vi "Parse Labels in Channel.vi"(8 "error in":errorcluster, 9 "channel #":u16, 10 "direction":T1, 11 "node in":refnum<k20>) -> (0 "error out":errorcluster, 3 "labels":T2[](array[typedef]))   [LabVIEW 2020, in "ARINC 429 Import.lvlib"]
uses:
  ARINC 429 Import.lvlib
  Encoding and Decoding/Encoding.ctl
  Encoding and Decoding/Encoding and Decoding.lvlib
  Read Tag Element (Boolean).vi
  Shared/Parameter Definition.ctl
  Shared/Direction.ctl
  Shared/VS Channel Definition for Parameter.ctl
  Shared/VS Channels Definition for Label.ctl
  Shared/Transfer Type.ctl
  Read Tag Element (String).vi
  Read Tag Element (U16).vi
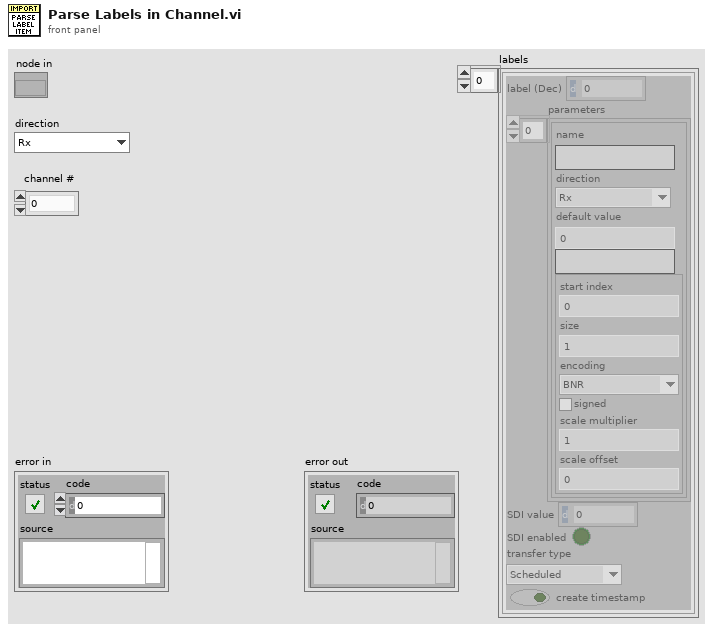
[diagram p1: front panel]
types:
  T1 = typedef "Direction.ctl" = enum16{"Rx", "Tx"}
  T2 = typedef "VS Channels Definition for Label.ctl" = cluster{"label (Dec)":u32, "parameters":T3[], "SDI value":u8, "SDI enabled":bool, "transfer type":T6, "create timestamp":bool}
  T3 = typedef "VS Channel Definition for Parameter.ctl" = cluster{"name":string, "direction":T1, "default value":dbl, "unit":string, "Parameter":T4}
  T4 = typedef "Parameter Definition.ctl" = cluster{"start index":i32, "size":i32, "encoding":T5, "signed":bool, "scale multiplier":dbl, "scale offset":dbl}
  T5 = typedef "Encoding and Decoding.lvlib/Encoding.ctl" = enum16{"BNR", "BCD", "Discrete"}
  T6 = typedef "Transfer Type.ctl" = enum16{"Scheduled", "Acyclic", "Block", "Strobe"}
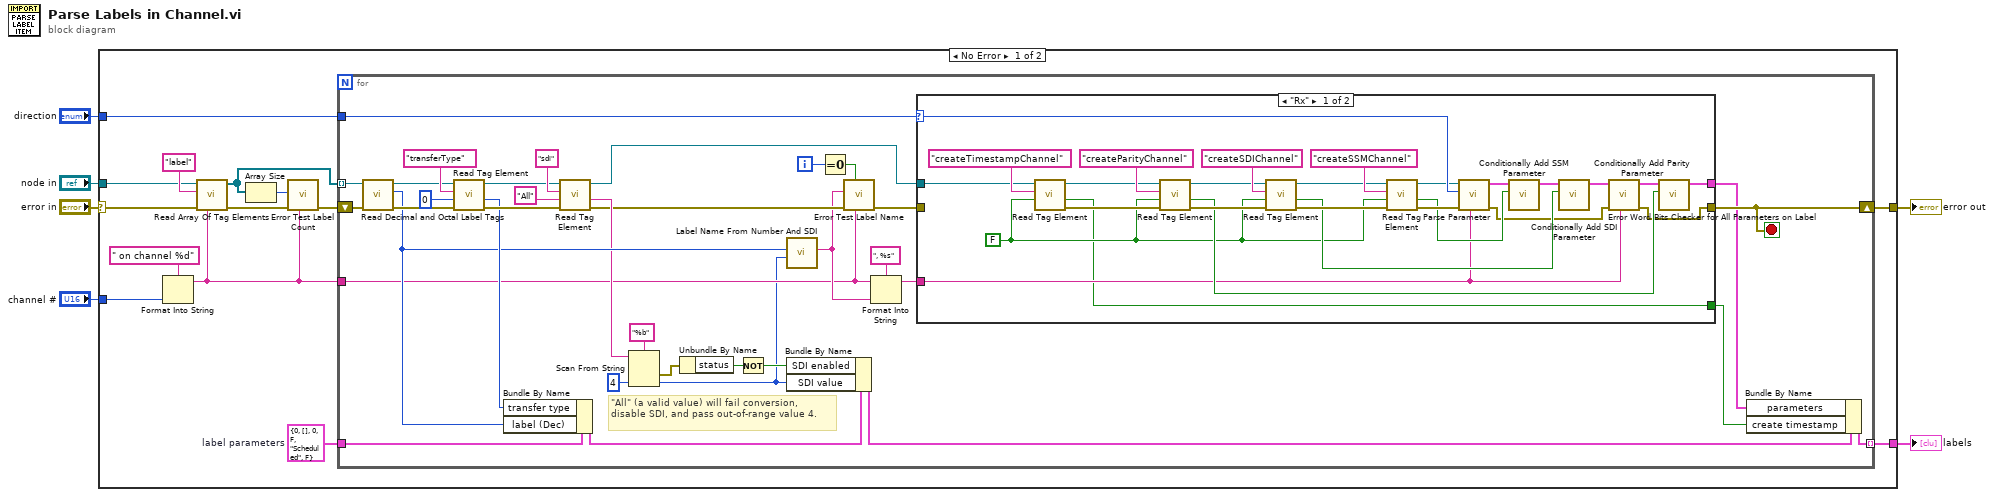
[diagram p0: block diagram]
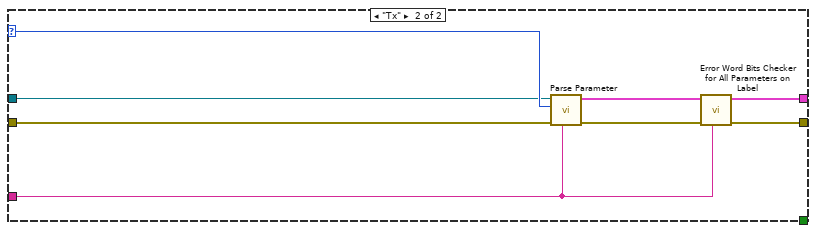
[diagram p2: hidden frame]
diagram:
  n1 = case shown="No Error" "error in" {
    selector: "error in" -> [w13 w92]
    tunnel: [w20 _] -> w6
    tunnel: "node in" -> [w16 _]
    tunnel: [w15 w92] -> w4
    tunnel: "direction" -> [w14 _]
    tunnel: "channel #" -> [w9 _]
    frame No Error {
      w11 = T2 {"label (Dec)"=0, "parameters"=[], "SDI value"=0, "SDI enabled"=FALSE, "transfer type"=enum."Scheduled", "create timestamp"=FALSE}  # label parameters
      n2 = Format Into String(format string=" on channel %d", w9) -> (resulting string=w10:string)  [unwired: 2 in, 1 out]
      n3 = call "Read Array Of Tag Elements.vi"("error text in"=w10, "error in"=w13, "tag name"="label" ("Tag Name"), "node in"=w16) -> ("error out"=w18:errorcluster, "array of elements"=w7:refnum<k20>[])  [unwired: 6 in]
      n4 = Array Size(array=w7) -> (size(s)=w8:i32)
      n5 = call "Error Test Label Count.vi"("error text in"=w10, "error in"=w18, "number of labels"=w8) -> ("error out"=w17:errorcluster)  [unwired: 8 in]
      n6 = for {
        shift-right: [w34] -> w15
        shift-left: w17 -> [w37]
        tunnel: [w48] -> w20 mode=indexing
        tunnel: w7 -> [w46] mode=indexing
        tunnel: w14 -> [w35]
        tunnel: w11 -> [w38]
        tunnel: w10 -> [w23]
        i -> [w26]
        stop <- w34 stop-if-true
        # "\"All\" (a valid value) will fail conversion, disable SDI, and pass out-of-range value 4."
        n7 = call "Read Decimal and Octal Label Tags.vi"("error in"=w37, "node in"=w46) -> ("error out"=w43:errorcluster, "label (Dec)"=w31:u32, "node out"=w44:refnum<k20>)  [unwired: 7 in]
        n8 = call-poly "Read Tag Element.vi"("error in"=w43, "default"=u16 0, "Tag Name"="transferType", "node in"=w44) -> ("error out"=w41:errorcluster, "value"=w39:u16, "node out"=w42:refnum<k20>)  [unwired: 5 in]
        n9 = Bundle By Name(cluster=w38, "transfer type"=w39, "label (Dec)"=w31) -> (w47:T2)
        n10 = call-poly "Read Tag Element.vi"("error in"=w41, "default"="All", "Tag Name"="sdi", "node in"=w42) -> ("error out"=w29:errorcluster, "value"=w30:string, "node out"=w27:refnum<k20>)  [unwired: 5 in]
        n11 = Scan From String(format string="%b", input string=w30, default 1=u8 4 ("default value 1")) -> (error out=w52:errorcluster, output 1=w22:u8)  [unwired: 2 in, 2 out]
        n12 = Unbundle By Name(w52) -> ("status"=w51:bool)
        n13 = Not(x=w51) -> (.not. x?=w50:bool)
        n14 = call "Label Name From Number And SDI.vi"("SDI value"=w22, "label (Dec)"=w31) -> ("label name"=w24:string)  [unwired: 9 in]
        n15 = Bundle By Name(cluster=w47, "SDI enabled"=w50, "SDI value"=w22) -> (w49:T2)
        n16 = Equal To 0?(x=w26) -> (x = 0?=w25:bool)
        n17 = call "Error Test Label Name.vi"("error text in"=w23, "reset (F)"=w25, "error in"=w29, "label name"=w24) -> ("error out"=w28:errorcluster)  [unwired: 7 in]
        n18 = Format Into String(format string=", %s", initial string=w23, w24) -> (resulting string=w33:string)  [unwired: 1 in, 1 out]
        n19 = case shown="\"Rx\"" w35 {
          selector: w35 -> [w77 w91]
          tunnel: [w64 w89] -> w34
          tunnel: w33 -> [w63 w84]
          tunnel: [w75 w88] -> w32
          tunnel: w27 -> [w61 w87]
          tunnel: w28 -> [_ w86]
          tunnel: [w57 _] -> w21
          frame "Rx" {
            w58 = FALSE
            n20 = call-poly "Read Tag Element.vi"("default"=w58, "Tag Name"="createTimestampChannel", "node in"=w61) -> ("error out"=w59:errorcluster, "value"=w57:bool, "node out"=w60:refnum<k20>)  [unwired: 6 in]
            n21 = call-poly "Read Tag Element.vi"("error in"=w59, "default"=w58, "Tag Name"="createParityChannel", "node in"=w60) -> ("error out"=w73:errorcluster, "value"=w67:bool, "node out"=w74:refnum<k20>)  [unwired: 5 in]
            n22 = call-poly "Read Tag Element.vi"("error in"=w73, "default"=w58, "Tag Name"="createSDIChannel", "node in"=w74) -> ("error out"=w79:errorcluster, "value"=w78:bool, "node out"=w80:refnum<k20>)  [unwired: 5 in]
            n23 = call-poly "Read Tag Element.vi"("error in"=w79, "default"=w58, "Tag Name"="createSSMChannel", "node in"=w80) -> ("error out"=w71:errorcluster, "value"=w66:bool, "node out"=w72:refnum<k20>)  [unwired: 5 in]
            n24 = call "Parse Parameter.vi"("error text in"=w63, "error in"=w71, "direction"=w77, "node in"=w72) -> ("error out"=w65:errorcluster, "parametesrs"=w70:T3[])  [unwired: 6 in]
            n25 = call "Conditionally Add SSM Parameter.vi"("create SSM (F)"=w66, "parameters in"=w70) -> ("parameters out"=w69:T3[])  [unwired: 9 in]
            n26 = call "Conditionally Add SDI Parameter.vi"("create SDI (F)"=w78, "parameters in"=w69) -> ("parameters out"=w68:T3[])  [unwired: 9 in]
            n27 = call "Error Word Bits Checker for All Parameters on Label.vi"("error text in"=w63, "error in"=w65, "parameters in"=w68) -> ("error out"=w64:errorcluster, "parameters out"=w76:T3[])  [unwired: 7 in]
            n28 = call "Conditionally Add Parity Parameter.vi"("create parity (F)"=w67, "parameters in"=w76) -> ("parameters out"=w75:T3[])  [unwired: 9 in]
          }
          frame "Tx" {
            n29 = call "Parse Parameter.vi"("error text in"=w84, "error in"=w86, "direction"=w91, "node in"=w87) -> ("error out"=w90:errorcluster, "parametesrs"=w85:T3[])  [unwired: 6 in]
            n30 = call "Error Word Bits Checker for All Parameters on Label.vi"("error text in"=w84, "error in"=w90, "parameters in"=w85) -> ("error out"=w89:errorcluster, "parameters out"=w88:T3[])  [unwired: 7 in]
          }
        }
        n31 = Bundle By Name(cluster=w49, "parameters"=w32, "create timestamp"=w21) -> (w48:T2)
      }
    }
    frame Error {
    }
  }
  "labels" <- w6
  "error out" <- w4
